vi "DataVIS_Read OLD .DAT Data.vi"(8 "error in (no error)":errorcluster, 11 "file path (use dialog)":path) -> (0 "error out":errorcluster, 3 "Array":T1(array[cluster]))   [LabVIEW 2016]
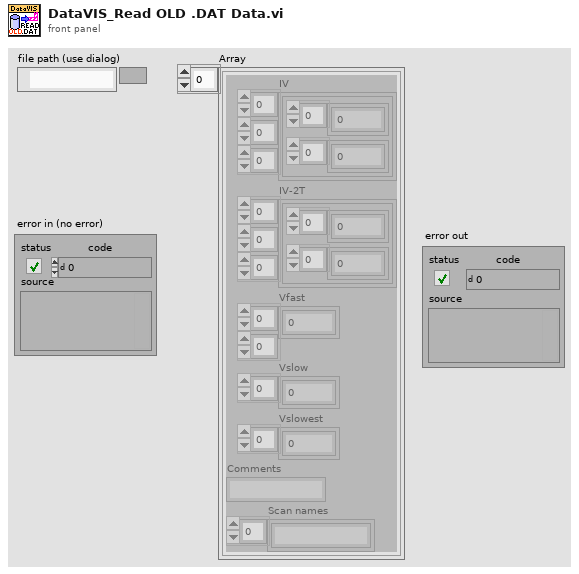
[diagram p1: front panel]
types:
  T1 = cluster{"IV":cluster{dbl[], dbl[]}[][][], "IV-2T":cluster{dbl[], dbl[]}[][][], "Vfast":dbl[][], "Vslow":dbl[], "Vslowest":dbl[], "Comments":string, "Scan names":string[]}[]
  T2 = cluster{"IV":cluster{dbl[], dbl[]}[][][], "IV-2T":cluster{dbl[], dbl[]}[][][], "Vfast":dbl[][], "Vslow":dbl[], "Vslowest":dbl[], "Comments":string, "Scan names":string[]}
  T3 = enum16{"open", "replace", "create", "open or create", "replace or create", "replace or create with confirmation"}
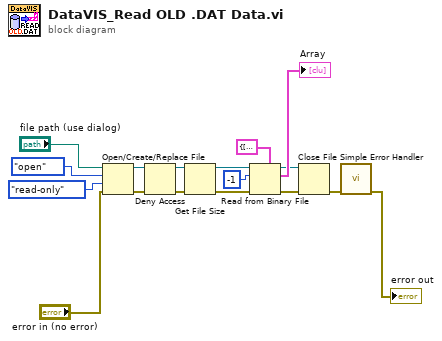
[diagram p0: block diagram]
diagram:
  n1 = Open/Create/Replace File(file path (use dialog)="file path (use dialog)", error in="error in (no error)", operation (0:open)=T3."open", access (0:read/write)=enum16{"read/write", "read-only", "write-only"}."read-only") -> (refnum out=w10:refnum<file>, error out=w9:errorcluster)  [unwired: 2 in, 1 out]
  n2 = Deny Access(4:w9, 7:w10) -> (0:w11:errorcluster, 3:w12:refnum<file>)  [unwired: 1 in]
  n3 = Get File Size(file=w12, error in=w11) -> (refnum out=w3:refnum<file>, 0:w7:errorcluster)  [unwired: 1 out]
  n4 = Read from Binary File(5:T2 {"IV"=[], "IV-2T"=[], "Vfast"=[], "Vslow"=[], "Vslowest"=[], "Comments"="", "Scan names"=[]} ("output cluster"), 8:w7, 10:-1 ("count (1)"), 11:w3) -> (0:w5:errorcluster, 2:→"Array":T1, 3:w4:refnum<file>)  [unwired: 2 in, 1 out]
  n5 = Close File(refnum=w4, error in=w5) -> (error out=w6:errorcluster)  [unwired: 1 out]
  n6 = call <vilib>:"Simple Error Handler.vi"("error in (no error)"=w6) -> ("error out"=→"error out":errorcluster)  [unwired: 4 in, 4 out]
